vi "Send Inline Buffer.vi"(8 "error in (no error)":errorcluster, 10 "Framework Inline Buffer":refnum<class "Buffer.lvclass">, 11 "Plugin Interface in":refnum<class "Plugin Interface.lvclass">) -> (0 "error out":errorcluster, 3 "Plugin Interface out":refnum<class "Plugin Interface.lvclass">)   [LabVIEW 2017, in "DSF Core.lvlib" / "Plugin Interface.lvclass"]
uses:
  Interfaces/Transceiver Interface/Plugin Interface.lvclass
  C:/Users/Admin/Desktop/Data Sharing Framework/Source/Core/Engine/Classes/Interfaces/Interface/Interface.lvclass
  Buffer/Buffer.lvclass
  C:/Program Files (x86)/National Instruments/LabVIEW 2017/vi.lib/NI/Memory Manager/Classes/Pointer/Pointer.lvclass
  Interfaces/Transceiver Interface/Command Data.ctl
  Interfaces/Transceiver Interface/Command.ctl
  Interfaces/Transceiver Interface/Command Parameters.ctl
  <vilib>/NI/Memory Manager/Classes/Pointer/Pointer.lvclass/Pointer.ctl
  Interfaces/Interface/Interface.lvclass/Interface.ctl
  Interfaces/Transceiver Interface/Response.ctl
  Interfaces/Transceiver Interface/Write Plugin Command.vi
  Interfaces/Interface/Write Command.vi
  Interfaces/Interface/Write RT FIFO.vi
  Interfaces/Dispatcher/Command Timeout.vi
  Interfaces/Transceiver Interface/Read Plugin Response.vi
  Interfaces/Dispatcher/Invalid Response.vi
  Interfaces/Dispatcher/Invalid Response Parameters.vi
  <vilib>/NI/Memory Manager/Classes/Pointer/Pointer.lvclass
  Interfaces/Interface/Interface.lvclass
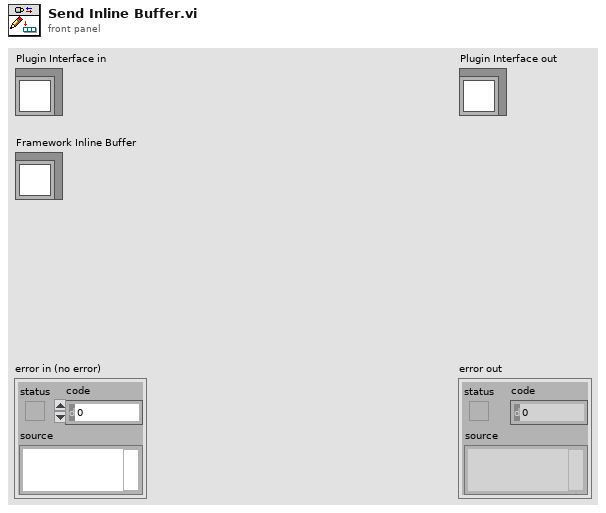
[diagram p1: front panel]
types:
  T1 = typedef "DSF Core.lvlib/Plugin Interface.lvclass/Command Data.ctl" = cluster{"Command":T2, "Parameters":T3}
  T2 = typedef "DSF Core.lvlib/Plugin Interface.lvclass/Command.ctl" = enum8{"Set Inline Buffer", "Rx", "Tx", "Shutdown"}
  T3 = typedef "DSF Core.lvlib/Plugin Interface.lvclass/Command Parameters.ctl" = cluster{"arg1":u64, "arg2":u64}
  T4 = typedef "DSF Core.lvlib/Plugin Interface.lvclass/Response.ctl" = enum8{"General Ack", "Shutting Down"}
  T5 = typedef "DSF Core.lvlib/Plugin Interface.lvclass/Response Data.ctl" = cluster{"Response":T4, "Parameters":T6}
  T6 = typedef "DSF Core.lvlib/Plugin Interface.lvclass/Response Parameters.ctl" = cluster{"arg1":u64, "arg2":u64}
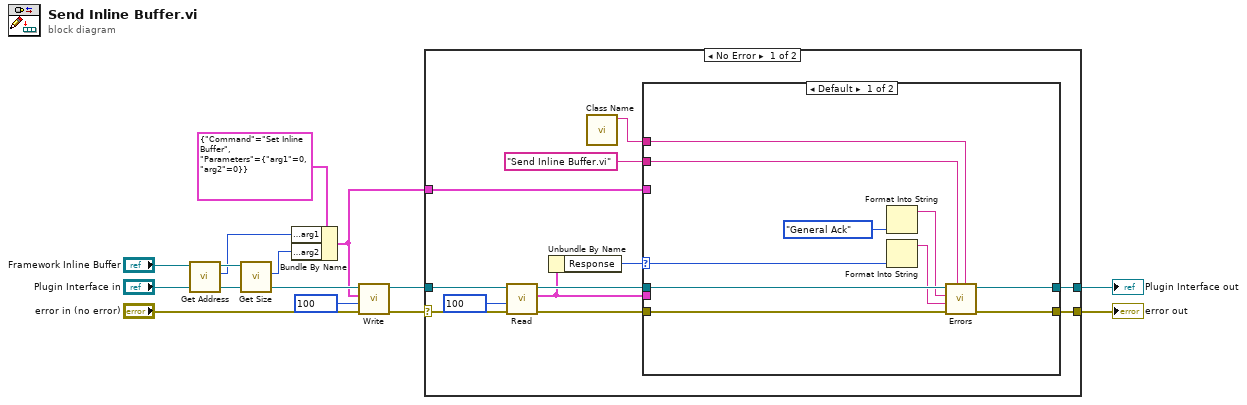
[diagram p0: block diagram]
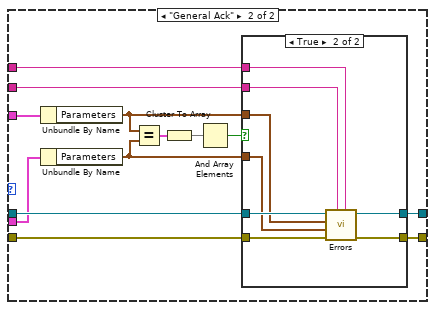
[diagram p2: hidden frame]
diagram:
  n1 = call <vilib>:"Get Address.vi"("Pointer in"="Framework Inline Buffer") -> ("address"=w7:u64, "Pointer out"=w9:refnum<class "Buffer.lvclass">)  [unwired: 9 in]
  n2 = call <vilib>:"Get Size.vi"("Pointer in"=w9) -> ("size"=w8:u64)  [unwired: 9 in, 1 out]
  n3 = Bundle By Name(cluster=T1 {"Command"=enum."Set Inline Buffer", "Parameters"={"arg1"=0, "arg2"=0}} ("command"), "Parameters.arg1"=w7, "Parameters.arg2"=w8) -> (w1:T1)
  n4 = call-poly "Write.vi"("error in (no error)"="error in (no error)", "timeout in ms (0)"=100, "command"=w1, "Plugin Interface in"="Plugin Interface in") -> ("error out"=w5:errorcluster, "Plugin Interface out"=w6:refnum<class "Plugin Interface.lvclass">)  [unwired: 6 in]
  n5 = case shown="No Error" w5 {
    selector: w5 -> [w22 w59]
    tunnel: w6 -> [w23 w60]
    tunnel: [w25 w59] -> w13
    tunnel: [w24 w60] -> w12
    tunnel: w1 -> [w16 _]
    frame No Error {
      n6 = call-poly "Read.vi"("error in (no error)"=w22, "timeout in ms (0)"=100, "Plugin Interface in"=w23) -> ("error out"=w20:errorcluster, "response"=w18:T5, "Plugin Interface out"=w21:refnum<class "Plugin Interface.lvclass">)  [unwired: 5 in, 1 out]
      n7 = Unbundle By Name(w18) -> ("Response"=w17:T4)
      n8 = call "Class Name.vi"() -> ("class name"=w15:string)  [unwired: 11 in]
      n9 = case shown="Default" w17 {
        selector: w17 -> [w28 _]
        tunnel: w20 -> [w34 w44]
        tunnel: [w33 w41] -> w25
        tunnel: w21 -> [w35 w45]
        tunnel: [w32 w42] -> w24
        tunnel: w18 -> [_ w43]
        tunnel: w16 -> [_ w48]
        tunnel: w15 -> [w26 w37]
        tunnel: "Send Inline Buffer.vi" ("error source vi name") -> [w27 w36]
        frame Default {
          n10 = Format Into String(Response."General Ack" ("x")) -> (resulting string=w30:string)  [unwired: 3 in, 1 out]
          n11 = Format Into String(w28) -> (resulting string=w29:string)  [unwired: 3 in, 1 out]
          n12 = call-poly "Errors.vi"("error source class name"=w26, "error source vi name"=w27, "error in (no error)"=w34, "actual response"=w29, "expected response"=w30, "Interface in"=w35) -> ("error out"=w33:errorcluster, "Interface out"=w32:refnum<class "Plugin Interface.lvclass">)  [unwired: 4 in]
        }
        frame "General Ack" {
          n13 = Unbundle By Name(w48) -> ("Parameters"=w39:T3)
          n14 = Unbundle By Name(w43) -> ("Parameters"=w38:T6)
          n15 = Equal?(x=w39, y=w38) -> (x = y?=w47:cluster{"arg1":bool, "arg2":bool})
          n16 = Cluster To Array(cluster=w47) -> (array=w46:bool[])
          n17 = And Array Elements(Boolean array=w46) -> (logical AND=w40:bool)
          n18 = case shown="True" w40 {
            tunnel: w45 -> [w50 w58]
            tunnel: w44 -> [w49 w57]
            tunnel: [w50 w56] -> w42
            tunnel: [w49 w55] -> w41
            tunnel: w39 -> [_ w54]
            tunnel: w38 -> [_ w53]
            tunnel: w37 -> [_ w52]
            tunnel: w36 -> [_ w51]
            frame False {
            }
            frame True {
              n19 = call-poly "Errors.vi"("error source class name"=w52, "error source vi name"=w51, "error in (no error)"=w57, "actual parameters"=w53, "expected parameters"=w54, "Interface in"=w58) -> ("error out"=w55:errorcluster, "Interface out"=w56:refnum<class "Plugin Interface.lvclass">)  [unwired: 4 in]
            }
          }
        }
      }
    }
    frame Error {
    }
  }
  "error out" <- w13
  "Plugin Interface out" <- w12
